vi "PRM - GetParameter.vi"(8 "error in (no error)":errorcluster, 11 "PRM":T1) -> (0 "error out":errorcluster, 3 "PRM OUT":T1, 5 "ParameterString":string)   [LabVIEW 2016]
doc: "Low Level function call. Converts LabVIEW enumeration to xiAPI parameter String."
uses:
  PRM_v2.ctl
  C:/Users/Ries Lab/Documents/Microscope Control from Sheng Account/Microscope-Control/Device Library/Cameras/Ximea/xiLIB_64bit/xiLIB/xiCamLib/API/x64/xiApi.NETX64.dll
  API/x64/xiApi.NETX64.dll
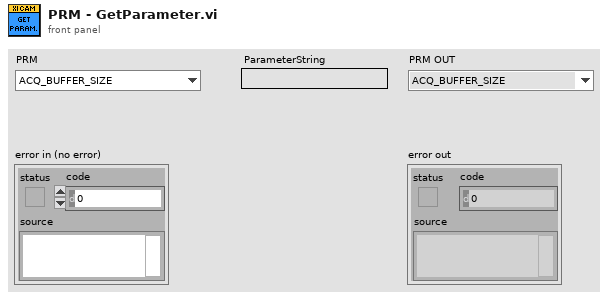
[diagram p1: front panel]
types:
  T1 = typedef "PRM_v2.ctl" = enum16{"ACQ_BUFFER_SIZE", "ACQ_FRAME_BURST_COUNT", "ACQ_TIMING_MODE", "ACQ_TRANSPORT_BUFFER_SIZE", "AE_MAX_LIMIT", "AEAG", "AEAG_LEVEL", "API_VERSION", "AG_MAX_LIMIT", "APPLY_CMS", "AUTO_BANDWIDTH_CALCULATION", "AUTO_WB", "AVAILABLE_BANDWIDTH", "AVAILABLE_BANDWIDTH_MAX", "AVAILABLE_BANDWIDTH_MIN", "BUFFER_POLICY", "BUFFERS_QUEUE_SIZE", "CC_MATRIX_00", "CC_MATRIX_01", "CC_MATRIX_02", "CC_MATRIX_03", "CC_MATRIX_10", "CC_MATRIX_11", "CC_MATRIX_12", "CC_MATRIX_13", "CC_MATRIX_20", "CC_MATRIX_21", "CC_MATRIX_22", "CC_MATRIX_23", "CC_MATRIX_30", "CC_MATRIX_31", "CC_MATRIX_32", "CC_MATRIX_33", "CHIP_TEMP", "CMS", "COLOR_FILTER_ARRAY", "COOLING", "DEBOUNCE_EN", "DEBOUNCE_POL", "DEBOUNCE_T0", "DEBOUNCE_T1", "DEBUG_LEVEL", "DEFAULT_CC_MATRIX", "DEVICE_INSTANCE_PATH", "DEVICE_MODEL_ID", "DEVICE_NAME", "DEVICE_SN", "DEVICE_TYPE", "DEVICE_USER_ID", "DOWNSAMPLING", "DOWNSAMPLING_TYPE", "DRV_VERSION", "EXP_PRIORITY", "EXPOSURE", "EXPOSURE_MAX", "EXPOSURE_MIN", "FFS_FILE_NAME", "FPGA1_VERSION", "FRAMERATE", "FRAMERATE_MAX", "FRAMERATE_MIN", "FREE_FFS_SIZE", "GAIN", "GAIN_MAX", "GAIN_MIN", "GAMMAC", "GAMMAY", "GPI_LEVEL", "GPI_MODE", "GPI_SELECTOR", "GPO_MODE", "GPO_SELECTOR", "HDR", "HDR_T1", "HDR_T2", "HEIGHT", "HEIGHT_MAX", "HEIGHT_MIN", "HOUSE_TEMP", "IMAGE_DATA_FORMAT", "IMAGE_IS_COLOR", "INPUT_CMS_PROFILE", "IS_COOLED", "IS_DEVICE_EXIST", "KNEEPOINT1", "KNEEPOINT2", "LED_MODE", "LED_SELECTOR", "LIMIT_BANDWIDTH", "LIMIT_BANDWIDTH_MAX", "LIMIT_BANDWIDTH_MIN", "LUT_EN", "LUT_INDEX", "LUT_INDEX_MAX", "LUT_INDEX_MIN", "LUT_VALUE", "LUT_VALUE_MAX", "LUT_VALUE_MIN", "MANUAL_WB", "MCU1_VERSION", "MCU2_VERSION", "OFFSET_X", "OFFSET_X_MAX", "OFFSET_X_MIN", "OFFSET_Y", "OFFSET_Y_MAX", "OFFSET_Y_MIN", "OUTPUT_CMS_PROFILE", "OUTPUT_DATA_BIT_DEPTH", "OUTPUT_DATA_PACKING", "READ_FILE_FFS", "RECENT_FRAME", "SENSOR_DATA_BIT_DEPTH", "SENSOR_MODE", "SENSOR_TAPS", "SHARPNESS", "SHUTTER_TYPE", "TARGET_TEMP", "TRG_DELAY", "TRG_SELECTOR", "TRG_SOFTWARE", "TRG_SOURCE", "USED_FFS_SIZE", "WB_KB", "WB_KG", "WB_KR", "WIDTH", "WIDTH_MAX", "WIDTH_MIN", "WRITE_FILE_FFS", "ACQ_BUFFER_SIZE_UNIT", "ACQ_TRANSPORT_BUFFER_COMMIT", "AEAG_ROI_HEIGHT", "AEAG_ROI_OFFSET_X", "AEAG_ROU_OFFSET_Y", "AEAG_ROI_WIDTH", "API_CONTEXT_LIST", "BINNING_HORIZONTAL", "BINNING_SELECTOR", "BINNING_VERTICAL", "COLUMN_FPN_CORRECTION", "COUNTER_SELECTOR", "COUNTER_VALUE", "DECIMATION_HORIZONTAL", "DECIMATION_SELECTOR", "DECIMATION_VERTICAL", "DEVICE_ID", "DEVICE_LOCATION_PATH", "DEVICE_MANIFEST", "DEVICE_RESET", "DEVICE_SENS_SN", "EXPOSURE_BURST_COUNT", "FFS_ACCESS_KEY", "GAIN_SELECTOR", "HW_REVISION", "IMAGE_BLACK_LEVEL", "IMAGE_DATA_BIT_DEPTH", "IMAGE_DATA_FORMAT_RGB32_ALPHA", "IMAGE_PAYLOAD_SIZE", "LENS_APERTURE_VALUE", "LENS_FEATURE", "LENS_FEATURE_SELECTOR", "LENS_FOCAL_LENGTH", "LENS_FOCUS_DISTANCE", "LENS_FOCUS_MOVE", "LENS_FOCUS_MOVEMENT_VALUE", "LENS_MODE", "OUTPUT_DATA_PACKING_TYPE", "SENSOR_CLOCK_FREQ_HZ", "SENSOR_CLOCK_FREQ_INDEX", "SENSOR_FEATURE_SELECTOR", "SENSOR_FEATURE_VALUE", "SENSOR_OUTPUT_CHANNEL_COUNT", "TRANSPORT_PIXEL_FORMAT", "TS_RST_MODE", "TS_RST_SOURCE", "SENS_DEFECTS_CORR_LIST_SELECTOR", "SENS_DEFECTS_CORR", "SENS_DEFECTS_CORR_LIST_CONTENT", "DEVICE_UNIT_SELECTOR", "DEVICE_UNIT_REGISTER_SELECTOR", "DEVICE_UNIT_REGISTER_VALUE"}
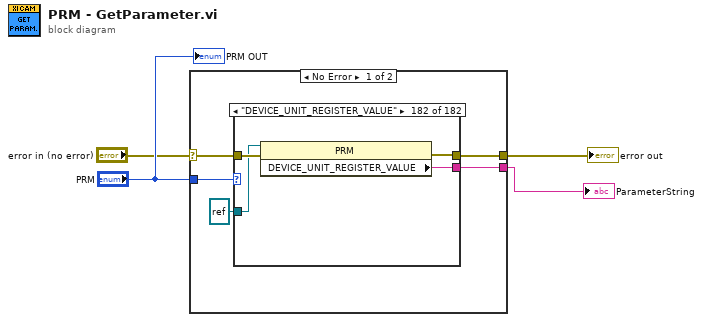
[diagram p0: block diagram]
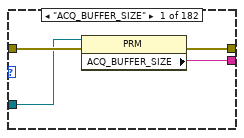
[diagram p2: hidden frame]
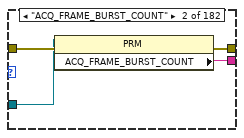
[diagram p3: hidden frame]
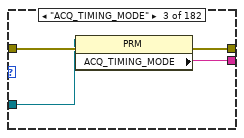
[diagram p4: hidden frame]
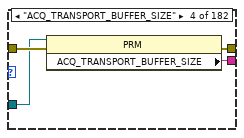
[diagram p5: hidden frame]
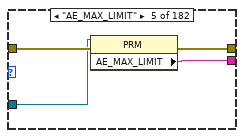
[diagram p6: hidden frame]
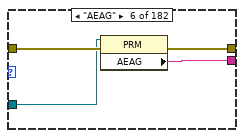
[diagram p7: hidden frame]
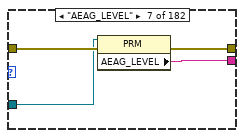
[diagram p8: hidden frame]
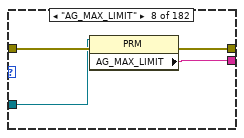
[diagram p9: hidden frame]
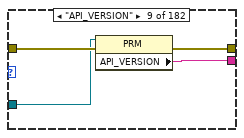
[diagram p10: hidden frame]
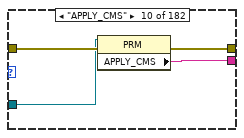
[diagram p11: hidden frame]
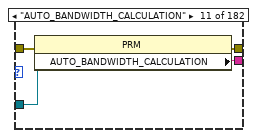
[diagram p12: hidden frame]
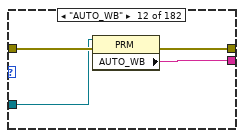
[diagram p13: hidden frame]
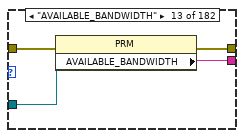
[diagram p14: hidden frame]
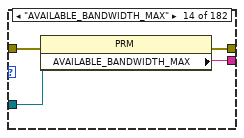
[diagram p15: hidden frame]
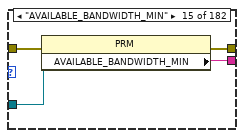
[diagram p16: hidden frame]
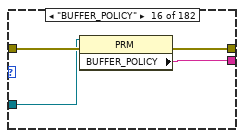
[diagram p17: hidden frame]
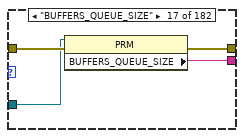
[diagram p18: hidden frame]
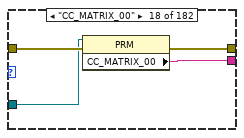
[diagram p19: hidden frame]
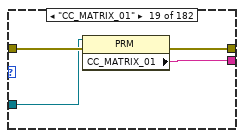
[diagram p20: hidden frame]
diagram:
  n1 = case shown="No Error" "error in (no error)" {
    selector: "error in (no error)" -> [w8 w738]
    tunnel: "PRM" -> [w9 _]
    tunnel: [w7 _] -> w1
    tunnel: [w6 w738] -> w2
    frame No Error {
      n2 = case shown="\"DEVICE_UNIT_REGISTER_VALUE\"" w9 {
        tunnel: w8 -> [w13 w17 w21 w25 w29 w33 w37 w41 w45 w49 w53 w57 w61 w65 w69 w73 w77 w81 w85 w89 w93 w97 w101 w105 w109 w113 w117 w121 w125 w129 w133 w137 w141 w145 w149 w153 w157 w161 w165 w169 w173 w177 w181 w185 w189 w193 w197 w201 w205 w209 w213 w217 w221 w225 w229 w233 w237 w241 w245 w249 w253 w257 w261 w265 w269 w273 w277 w281 w285 w289 w293 w297 w301 w305 w309 w313 w317 w321 w325 w329 w333 w337 w341 w345 w349 w353 w357 w361 w365 w369 w373 w377 w381 w385 w389 w393 w397 w401 w405 w409 w413 w417 w421 w425 w429 w433 w437 w441 w445 w449 w453 w457 w461 w465 w469 w473 w477 w481 w485 w489 w493 w497 w501 w505 w509 w513 w517 w521 w525 w529 w532 w536 w540 w544 w548 w552 w556 w560 w564 w568 w572 w576 w580 w584 w588 w592 w596 w600 w604 w608 w612 w616 w620 w624 w628 w632 w636 w640 w644 w648 w652 w656 w660 w664 w668 w672 w676 w680 w684 w688 w692 w696 w700 w704 w708 w712 w715 w721 w725 w729 w733 w737]
        tunnel: [w12 w16 w20 w24 w28 w32 w36 w40 w44 w48 w52 w56 w60 w64 w68 w72 w76 w80 w84 w88 w92 w96 w100 w104 w108 w112 w116 w120 w124 w128 w132 w136 w140 w144 w148 w152 w156 w160 w164 w168 w172 w176 w180 w184 w188 w192 w196 w200 w204 w208 w212 w216 w220 w224 w228 w232 w236 w240 w244 w248 w252 w256 w260 w264 w268 w272 w276 w280 w284 w288 w292 w296 w300 w304 w308 w312 w316 w320 w324 w328 w332 w336 w340 w344 w348 w352 w356 w360 w364 w368 w372 w376 w380 w384 w388 w392 w396 w400 w404 w408 w412 w416 w420 w424 w428 w432 w436 w440 w444 w448 w452 w456 w460 w464 w468 w472 w476 w480 w484 w488 w492 w496 w500 w504 w508 w512 w516 w520 w524 w528 w530 w534 w538 w542 w546 w550 w554 w558 w562 w566 w570 w574 w578 w582 w586 w590 w594 w598 w602 w606 w610 w614 w618 w622 w626 w630 w634 w638 w642 w646 w650 w654 w658 w662 w666 w670 w674 w678 w682 w686 w690 w694 w698 w702 w706 w710 w717 w719 w723 w726 w730 w734] -> w7
        tunnel: [w11 w15 w19 w23 w27 w31 w35 w39 w43 w47 w51 w55 w59 w63 w67 w71 w75 w79 w83 w87 w91 w95 w99 w103 w107 w111 w115 w119 w123 w127 w131 w135 w139 w143 w147 w151 w155 w159 w163 w167 w171 w175 w179 w183 w187 w191 w195 w199 w203 w207 w211 w215 w219 w223 w227 w231 w235 w239 w243 w247 w251 w255 w259 w263 w267 w271 w275 w279 w283 w287 w291 w295 w299 w303 w307 w311 w315 w319 w323 w327 w331 w335 w339 w343 w347 w351 w355 w359 w363 w367 w371 w375 w379 w383 w387 w391 w395 w399 w403 w407 w411 w415 w419 w423 w427 w431 w435 w439 w443 w447 w451 w455 w459 w463 w467 w471 w475 w479 w483 w487 w491 w495 w499 w503 w507 w511 w515 w519 w523 w527 w531 w535 w539 w543 w547 w551 w555 w559 w563 w567 w571 w575 w579 w583 w587 w591 w595 w599 w603 w607 w611 w615 w619 w623 w627 w631 w635 w639 w643 w647 w651 w655 w659 w663 w667 w671 w675 w679 w683 w687 w691 w695 w699 w703 w707 w711 w716 w720 w724 w727 w731 w735] -> w6
        tunnel: refnum<k24> refnum ("reference") -> [w10 w14 w18 w22 w26 w30 w34 w38 w42 w46 w50 w54 w58 w62 w66 w70 w74 w78 w82 w86 w90 w94 w98 w102 w106 w110 w114 w118 w122 w126 w130 w134 w138 w142 w146 w150 w154 w158 w162 w166 w170 w174 w178 w182 w186 w190 w194 w198 w202 w206 w210 w214 w218 w222 w226 w230 w234 w238 w242 w246 w250 w254 w258 w262 w266 w270 w274 w278 w282 w286 w290 w294 w298 w302 w306 w310 w314 w318 w322 w326 w330 w334 w338 w342 w346 w350 w354 w358 w362 w366 w370 w374 w378 w382 w386 w390 w394 w398 w402 w406 w410 w414 w418 w422 w426 w430 w434 w438 w442 w446 w450 w454 w458 w462 w466 w470 w474 w478 w482 w486 w490 w494 w498 w502 w506 w510 w514 w518 w522 w526 w533 w537 w541 w545 w549 w553 w557 w561 w565 w569 w573 w577 w581 w585 w589 w593 w597 w601 w605 w609 w613 w617 w621 w625 w629 w633 w637 w641 w645 w649 w653 w657 w661 w665 w669 w673 w677 w681 w685 w689 w693 w697 w701 w705 w709 w713 w714 w718 w722 w728 w732 w736]
        frame "ACQ_BUFFER_SIZE" {
          n3 = property class="PRM"(reference=w10, error in=w13) -> (error out=w11:errorcluster, "ACQ_BUFFER_SIZE"=w12:string)  [unwired: 1 out]
        }
        frame "ACQ_FRAME_BURST_COUNT" {
          n4 = property class="PRM"(reference=w14, error in=w17) -> (error out=w15:errorcluster, "ACQ_FRAME_BURST_COUNT"=w16:string)  [unwired: 1 out]
        }
        frame "ACQ_TIMING_MODE" {
          n5 = property class="PRM"(reference=w18, error in=w21) -> (error out=w19:errorcluster, "ACQ_TIMING_MODE"=w20:string)  [unwired: 1 out]
        }
        frame "ACQ_TRANSPORT_BUFFER_SIZE" {
          n6 = property class="PRM"(reference=w22, error in=w25) -> (error out=w23:errorcluster, "ACQ_TRANSPORT_BUFFER_SIZE"=w24:string)  [unwired: 1 out]
        }
        frame "AE_MAX_LIMIT" {
          n7 = property class="PRM"(reference=w26, error in=w29) -> (error out=w27:errorcluster, "AE_MAX_LIMIT"=w28:string)  [unwired: 1 out]
        }
        frame "AEAG" {
          n8 = property class="PRM"(reference=w30, error in=w33) -> (error out=w31:errorcluster, "AEAG"=w32:string)  [unwired: 1 out]
        }
        frame "AEAG_LEVEL" {
          n9 = property class="PRM"(reference=w34, error in=w37) -> (error out=w35:errorcluster, "AEAG_LEVEL"=w36:string)  [unwired: 1 out]
        }
        frame "AG_MAX_LIMIT" {
          n10 = property class="PRM"(reference=w38, error in=w41) -> (error out=w39:errorcluster, "AG_MAX_LIMIT"=w40:string)  [unwired: 1 out]
        }
        frame "API_VERSION" {
          n11 = property class="PRM"(reference=w42, error in=w45) -> (error out=w43:errorcluster, "API_VERSION"=w44:string)  [unwired: 1 out]
        }
        frame "APPLY_CMS" {
          n12 = property class="PRM"(reference=w46, error in=w49) -> (error out=w47:errorcluster, "APPLY_CMS"=w48:string)  [unwired: 1 out]
        }
        frame "AUTO_BANDWIDTH_CALCULATION" {
          n13 = property class="PRM"(reference=w50, error in=w53) -> (error out=w51:errorcluster, "AUTO_BANDWIDTH_CALCULATION"=w52:string)  [unwired: 1 out]
        }
        frame "AUTO_WB" {
          n14 = property class="PRM"(reference=w54, error in=w57) -> (error out=w55:errorcluster, "AUTO_WB"=w56:string)  [unwired: 1 out]
        }
        frame "AVAILABLE_BANDWIDTH" {
          n15 = property class="PRM"(reference=w58, error in=w61) -> (error out=w59:errorcluster, "AVAILABLE_BANDWIDTH"=w60:string)  [unwired: 1 out]
        }
        frame "AVAILABLE_BANDWIDTH_MAX" {
          n16 = property class="PRM"(reference=w62, error in=w65) -> (error out=w63:errorcluster, "AVAILABLE_BANDWIDTH_MAX"=w64:string)  [unwired: 1 out]
        }
        frame "AVAILABLE_BANDWIDTH_MIN" {
          n17 = property class="PRM"(reference=w66, error in=w69) -> (error out=w67:errorcluster, "AVAILABLE_BANDWIDTH_MIN"=w68:string)  [unwired: 1 out]
        }
        frame "BUFFER_POLICY" {
          n18 = property class="PRM"(reference=w70, error in=w73) -> (error out=w71:errorcluster, "BUFFER_POLICY"=w72:string)  [unwired: 1 out]
        }
        frame "BUFFERS_QUEUE_SIZE" {
          n19 = property class="PRM"(reference=w74, error in=w77) -> (error out=w75:errorcluster, "BUFFERS_QUEUE_SIZE"=w76:string)  [unwired: 1 out]
        }
        frame "CC_MATRIX_00" {
          n20 = property class="PRM"(reference=w78, error in=w81) -> (error out=w79:errorcluster, "CC_MATRIX_00"=w80:string)  [unwired: 1 out]
        }
        frame "CC_MATRIX_01" {
          n21 = property class="PRM"(reference=w82, error in=w85) -> (error out=w83:errorcluster, "CC_MATRIX_01"=w84:string)  [unwired: 1 out]
        }
        frame "CC_MATRIX_02" {
          n22 = property class="PRM"(reference=w86, error in=w89) -> (error out=w87:errorcluster, "CC_MATRIX_02"=w88:string)  [unwired: 1 out]
        }
        frame "CC_MATRIX_03" {
          n23 = property class="PRM"(reference=w90, error in=w93) -> (error out=w91:errorcluster, "CC_MATRIX_03"=w92:string)  [unwired: 1 out]
        }
        frame "CC_MATRIX_10" {
          n24 = property class="PRM"(reference=w94, error in=w97) -> (error out=w95:errorcluster, "CC_MATRIX_10"=w96:string)  [unwired: 1 out]
        }
        frame "CC_MATRIX_11" {
          n25 = property class="PRM"(reference=w98, error in=w101) -> (error out=w99:errorcluster, "CC_MATRIX_11"=w100:string)  [unwired: 1 out]
        }
        frame "CC_MATRIX_12" {
          n26 = property class="PRM"(reference=w102, error in=w105) -> (error out=w103:errorcluster, "CC_MATRIX_12"=w104:string)  [unwired: 1 out]
        }
        frame "CC_MATRIX_13" {
          n27 = property class="PRM"(reference=w106, error in=w109) -> (error out=w107:errorcluster, "CC_MATRIX_13"=w108:string)  [unwired: 1 out]
        }
        frame "CC_MATRIX_20" {
          n28 = property class="PRM"(reference=w110, error in=w113) -> (error out=w111:errorcluster, "CC_MATRIX_20"=w112:string)  [unwired: 1 out]
        }
        frame "CC_MATRIX_21" {
          n29 = property class="PRM"(reference=w114, error in=w117) -> (error out=w115:errorcluster, "CC_MATRIX_21"=w116:string)  [unwired: 1 out]
        }
        frame "CC_MATRIX_22" {
          n30 = property class="PRM"(reference=w118, error in=w121) -> (error out=w119:errorcluster, "CC_MATRIX_22"=w120:string)  [unwired: 1 out]
        }
        frame "CC_MATRIX_23" {
          n31 = property class="PRM"(reference=w122, error in=w125) -> (error out=w123:errorcluster, "CC_MATRIX_23"=w124:string)  [unwired: 1 out]
        }
        frame "CC_MATRIX_30" {
          n32 = property class="PRM"(reference=w126, error in=w129) -> (error out=w127:errorcluster, "CC_MATRIX_30"=w128:string)  [unwired: 1 out]
        }
        frame "CC_MATRIX_31" {
          n33 = property class="PRM"(reference=w130, error in=w133) -> (error out=w131:errorcluster, "CC_MATRIX_31"=w132:string)  [unwired: 1 out]
        }
        frame "CC_MATRIX_32" {
          n34 = property class="PRM"(reference=w134, error in=w137) -> (error out=w135:errorcluster, "CC_MATRIX_32"=w136:string)  [unwired: 1 out]
        }
        frame "CC_MATRIX_33" {
          n35 = property class="PRM"(reference=w138, error in=w141) -> (error out=w139:errorcluster, "CC_MATRIX_33"=w140:string)  [unwired: 1 out]
        }
        frame "CHIP_TEMP" {
          n36 = property class="PRM"(reference=w142, error in=w145) -> (error out=w143:errorcluster, "CHIP_TEMP"=w144:string)  [unwired: 1 out]
        }
        frame "CMS" {
          n37 = property class="PRM"(reference=w146, error in=w149) -> (error out=w147:errorcluster, "CMS"=w148:string)  [unwired: 1 out]
        }
        frame "COLOR_FILTER_ARRAY" {
          n38 = property class="PRM"(reference=w150, error in=w153) -> (error out=w151:errorcluster, "COLOR_FILTER_ARRAY"=w152:string)  [unwired: 1 out]
        }
        frame "COOLING" {
          n39 = property class="PRM"(reference=w154, error in=w157) -> (error out=w155:errorcluster, "COOLING"=w156:string)  [unwired: 1 out]
        }
        frame "DEBOUNCE_EN" {
          n40 = property class="PRM"(reference=w158, error in=w161) -> (error out=w159:errorcluster, "DEBOUNCE_EN"=w160:string)  [unwired: 1 out]
        }
        frame "DEBOUNCE_POL" {
          n41 = property class="PRM"(reference=w162, error in=w165) -> (error out=w163:errorcluster, "DEBOUNCE_POL"=w164:string)  [unwired: 1 out]
        }
        frame "DEBOUNCE_T0" {
          n42 = property class="PRM"(reference=w166, error in=w169) -> (error out=w167:errorcluster, "DEBOUNCE_T0"=w168:string)  [unwired: 1 out]
        }
        frame "DEBOUNCE_T1" {
          n43 = property class="PRM"(reference=w170, error in=w173) -> (error out=w171:errorcluster, "DEBOUNCE_T1"=w172:string)  [unwired: 1 out]
        }
        frame "DEBUG_LEVEL" {
          n44 = property class="PRM"(reference=w174, error in=w177) -> (error out=w175:errorcluster, "DEBUG_LEVEL"=w176:string)  [unwired: 1 out]
        }
        frame "DEFAULT_CC_MATRIX" {
          n45 = property class="PRM"(reference=w178, error in=w181) -> (error out=w179:errorcluster, "DEFAULT_CC_MATRIX"=w180:string)  [unwired: 1 out]
        }
        frame "DEVICE_INSTANCE_PATH" {
          n46 = property class="PRM"(reference=w182, error in=w185) -> (error out=w183:errorcluster, "DEVICE_INSTANCE_PATH"=w184:string)  [unwired: 1 out]
        }
        frame "DEVICE_MODEL_ID" {
          n47 = property class="PRM"(reference=w186, error in=w189) -> (error out=w187:errorcluster, "DEVICE_MODEL_ID"=w188:string)  [unwired: 1 out]
        }
        frame "DEVICE_NAME" {
          n48 = property class="PRM"(reference=w190, error in=w193) -> (error out=w191:errorcluster, "DEVICE_NAME"=w192:string)  [unwired: 1 out]
        }
        frame "DEVICE_SN" {
          n49 = property class="PRM"(reference=w194, error in=w197) -> (error out=w195:errorcluster, "DEVICE_SN"=w196:string)  [unwired: 1 out]
        }
        frame "DEVICE_TYPE" {
          n50 = property class="PRM"(reference=w198, error in=w201) -> (error out=w199:errorcluster, "DEVICE_TYPE"=w200:string)  [unwired: 1 out]
        }
        frame "DEVICE_USER_ID" {
          n51 = property class="PRM"(reference=w202, error in=w205) -> (error out=w203:errorcluster, "DEVICE_USER_ID"=w204:string)  [unwired: 1 out]
        }
        frame "DOWNSAMPLING" {
          n52 = property class="PRM"(reference=w206, error in=w209) -> (error out=w207:errorcluster, "DOWNSAMPLING"=w208:string)  [unwired: 1 out]
        }
        frame "DOWNSAMPLING_TYPE" {
          n53 = property class="PRM"(reference=w210, error in=w213) -> (error out=w211:errorcluster, "DOWNSAMPLING_TYPE"=w212:string)  [unwired: 1 out]
        }
        frame "DRV_VERSION" {
          n54 = property class="PRM"(reference=w214, error in=w217) -> (error out=w215:errorcluster, "DRV_VERSION"=w216:string)  [unwired: 1 out]
        }
        frame "EXP_PRIORITY" {
          n55 = property class="PRM"(reference=w218, error in=w221) -> (error out=w219:errorcluster, "EXP_PRIORITY"=w220:string)  [unwired: 1 out]
        }
        frame "EXPOSURE" {
          n56 = property class="PRM"(reference=w222, error in=w225) -> (error out=w223:errorcluster, "EXPOSURE"=w224:string)  [unwired: 1 out]
        }
        frame "EXPOSURE_MAX" {
          n57 = property class="PRM"(reference=w226, error in=w229) -> (error out=w227:errorcluster, "EXPOSURE_MAX"=w228:string)  [unwired: 1 out]
        }
        frame "EXPOSURE_MIN" {
          n58 = property class="PRM"(reference=w230, error in=w233) -> (error out=w231:errorcluster, "EXPOSURE_MIN"=w232:string)  [unwired: 1 out]
        }
        frame "FFS_FILE_NAME" {
          n59 = property class="PRM"(reference=w234, error in=w237) -> (error out=w235:errorcluster, "FFS_FILE_NAME"=w236:string)  [unwired: 1 out]
        }
        frame "FPGA1_VERSION" {
          n60 = property class="PRM"(reference=w238, error in=w241) -> (error out=w239:errorcluster, "FPGA1_VERSION"=w240:string)  [unwired: 1 out]
        }
        frame "FRAMERATE" {
          n61 = property class="PRM"(reference=w242, error in=w245) -> (error out=w243:errorcluster, "FRAMERATE"=w244:string)  [unwired: 1 out]
        }
        frame "FRAMERATE_MAX" {
          n62 = property class="PRM"(reference=w246, error in=w249) -> (error out=w247:errorcluster, "FRAMERATE_MAX"=w248:string)  [unwired: 1 out]
        }
        frame "FRAMERATE_MIN" {
          n63 = property class="PRM"(reference=w250, error in=w253) -> (error out=w251:errorcluster, "FRAMERATE_MIN"=w252:string)  [unwired: 1 out]
        }
        frame "FREE_FFS_SIZE" {
          n64 = property class="PRM"(reference=w254, error in=w257) -> (error out=w255:errorcluster, "FREE_FFS_SIZE"=w256:string)  [unwired: 1 out]
        }
        frame "GAIN" {
          n65 = property class="PRM"(reference=w258, error in=w261) -> (error out=w259:errorcluster, "GAIN"=w260:string)  [unwired: 1 out]
        }
        frame "GAIN_MAX" {
          n66 = property class="PRM"(reference=w262, error in=w265) -> (error out=w263:errorcluster, "GAIN_MAX"=w264:string)  [unwired: 1 out]
        }
        frame "GAIN_MIN" {
          n67 = property class="PRM"(reference=w266, error in=w269) -> (error out=w267:errorcluster, "GAIN_MIN"=w268:string)  [unwired: 1 out]
        }
        frame "GAMMAC" {
          n68 = property class="PRM"(reference=w270, error in=w273) -> (error out=w271:errorcluster, "GAMMAC"=w272:string)  [unwired: 1 out]
        }
        frame "GAMMAY" {
          n69 = property class="PRM"(reference=w274, error in=w277) -> (error out=w275:errorcluster, "GAMMAY"=w276:string)  [unwired: 1 out]
        }
        frame "GPI_LEVEL" {
          n70 = property class="PRM"(reference=w278, error in=w281) -> (error out=w279:errorcluster, "GPI_LEVEL"=w280:string)  [unwired: 1 out]
        }
        frame "GPI_MODE" {
          n71 = property class="PRM"(reference=w282, error in=w285) -> (error out=w283:errorcluster, "GPI_MODE"=w284:string)  [unwired: 1 out]
        }
        frame "GPI_SELECTOR" {
          n72 = property class="PRM"(reference=w286, error in=w289) -> (error out=w287:errorcluster, "GPI_SELECTOR"=w288:string)  [unwired: 1 out]
        }
        frame "GPO_MODE" {
          n73 = property class="PRM"(reference=w290, error in=w293) -> (error out=w291:errorcluster, "GPO_MODE"=w292:string)  [unwired: 1 out]
        }
        frame "GPO_SELECTOR" {
          n74 = property class="PRM"(reference=w294, error in=w297) -> (error out=w295:errorcluster, "GPO_SELECTOR"=w296:string)  [unwired: 1 out]
        }
        frame "HDR" {
          n75 = property class="PRM"(reference=w298, error in=w301) -> (error out=w299:errorcluster, "HDR"=w300:string)  [unwired: 1 out]
        }
        frame "HDR_T1" {
          n76 = property class="PRM"(reference=w302, error in=w305) -> (error out=w303:errorcluster, "HDR_T1"=w304:string)  [unwired: 1 out]
        }
        frame "HDR_T2" {
          n77 = property class="PRM"(reference=w306, error in=w309) -> (error out=w307:errorcluster, "HDR_T2"=w308:string)  [unwired: 1 out]
        }
        frame "HEIGHT" {
          n78 = property class="PRM"(reference=w310, error in=w313) -> (error out=w311:errorcluster, "HEIGHT"=w312:string)  [unwired: 1 out]
        }
        frame "HEIGHT_MAX" {
          n79 = property class="PRM"(reference=w314, error in=w317) -> (error out=w315:errorcluster, "HEIGHT_MAX"=w316:string)  [unwired: 1 out]
        }
        frame "HEIGHT_MIN" {
          n80 = property class="PRM"(reference=w318, error in=w321) -> (error out=w319:errorcluster, "HEIGHT_MIN"=w320:string)  [unwired: 1 out]
        }
        frame "HOUSE_TEMP" {
          n81 = property class="PRM"(reference=w322, error in=w325) -> (error out=w323:errorcluster, "HOUS_TEMP"=w324:string)  [unwired: 1 out]
        }
        frame "IMAGE_DATA_FORMAT" {
          n82 = property class="PRM"(reference=w326, error in=w329) -> (error out=w327:errorcluster, "IMAGE_DATA_FORMAT"=w328:string)  [unwired: 1 out]
        }
        frame "IMAGE_IS_COLOR" {
          n83 = property class="PRM"(reference=w330, error in=w333) -> (error out=w331:errorcluster, "IMAGE_IS_COLOR"=w332:string)  [unwired: 1 out]
        }
        frame "INPUT_CMS_PROFILE" {
          n84 = property class="PRM"(reference=w334, error in=w337) -> (error out=w335:errorcluster, "INPUT_CMS_PROFILE"=w336:string)  [unwired: 1 out]
        }
        frame "IS_COOLED" {
          n85 = property class="PRM"(reference=w338, error in=w341) -> (error out=w339:errorcluster, "IS_COOLED"=w340:string)  [unwired: 1 out]
        }
        frame "IS_DEVICE_EXIST" {
          n86 = property class="PRM"(reference=w342, error in=w345) -> (error out=w343:errorcluster, "IS_DEVICE_EXIST"=w344:string)  [unwired: 1 out]
        }
        frame "KNEEPOINT1" {
          n87 = property class="PRM"(reference=w346, error in=w349) -> (error out=w347:errorcluster, "KNEEPOINT1"=w348:string)  [unwired: 1 out]
        }
        frame "KNEEPOINT2" {
          n88 = property class="PRM"(reference=w350, error in=w353) -> (error out=w351:errorcluster, "KNEEPOINT2"=w352:string)  [unwired: 1 out]
        }
        frame "LED_MODE" {
          n89 = property class="PRM"(reference=w354, error in=w357) -> (error out=w355:errorcluster, "LED_MODE"=w356:string)  [unwired: 1 out]
        }
        frame "LED_SELECTOR" {
          n90 = property class="PRM"(reference=w358, error in=w361) -> (error out=w359:errorcluster, "LED_SELECTOR"=w360:string)  [unwired: 1 out]
        }
        frame "LIMIT_BANDWIDTH" {
          n91 = property class="PRM"(reference=w362, error in=w365) -> (error out=w363:errorcluster, "LIMIT_BANDWIDTH"=w364:string)  [unwired: 1 out]
        }
        frame "LIMIT_BANDWIDTH_MAX" {
          n92 = property class="PRM"(reference=w366, error in=w369) -> (error out=w367:errorcluster, "LIMIT_BANDWIDTH_MAX"=w368:string)  [unwired: 1 out]
        }
        frame "LIMIT_BANDWIDTH_MIN" {
          n93 = property class="PRM"(reference=w370, error in=w373) -> (error out=w371:errorcluster, "LIMIT_BANDWIDTH_MIN"=w372:string)  [unwired: 1 out]
        }
        frame "LUT_EN" {
          n94 = property class="PRM"(reference=w374, error in=w377) -> (error out=w375:errorcluster, "LUT_EN"=w376:string)  [unwired: 1 out]
        }
        frame "LUT_INDEX" {
          n95 = property class="PRM"(reference=w378, error in=w381) -> (error out=w379:errorcluster, "LUT_INDEX"=w380:string)  [unwired: 1 out]
        }
        frame "LUT_INDEX_MAX" {
          n96 = property class="PRM"(reference=w382, error in=w385) -> (error out=w383:errorcluster, "LUT_INDEX_MAX"=w384:string)  [unwired: 1 out]
        }
        frame "LUT_INDEX_MIN" {
          n97 = property class="PRM"(reference=w386, error in=w389) -> (error out=w387:errorcluster, "LUT_INDEX_MIN"=w388:string)  [unwired: 1 out]
        }
        frame "LUT_VALUE" {
          n98 = property class="PRM"(reference=w390, error in=w393) -> (error out=w391:errorcluster, "LUT_VALUE"=w392:string)  [unwired: 1 out]
        }
        frame "LUT_VALUE_MAX" {
          n99 = property class="PRM"(reference=w394, error in=w397) -> (error out=w395:errorcluster, "LUT_VALUE_MAX"=w396:string)  [unwired: 1 out]
        }
        frame "LUT_VALUE_MIN" {
          n100 = property class="PRM"(reference=w398, error in=w401) -> (error out=w399:errorcluster, "LUT_VALUE_MIN"=w400:string)  [unwired: 1 out]
        }
        frame "MANUAL_WB" {
          n101 = property class="PRM"(reference=w402, error in=w405) -> (error out=w403:errorcluster, "MANUAL_WB"=w404:string)  [unwired: 1 out]
        }
        frame "MCU1_VERSION" {
          n102 = property class="PRM"(reference=w406, error in=w409) -> (error out=w407:errorcluster, "MCU1_VERSION"=w408:string)  [unwired: 1 out]
        }
        frame "MCU2_VERSION" {
          n103 = property class="PRM"(reference=w410, error in=w413) -> (error out=w411:errorcluster, "MCU2_VERSION"=w412:string)  [unwired: 1 out]
        }
        frame "OFFSET_X" {
          n104 = property class="PRM"(reference=w414, error in=w417) -> (error out=w415:errorcluster, "OFFSET_X"=w416:string)  [unwired: 1 out]
        }
        frame "OFFSET_X_MAX" {
          n105 = property class="PRM"(reference=w418, error in=w421) -> (error out=w419:errorcluster, "OFFSET_X_MAX"=w420:string)  [unwired: 1 out]
        }
        frame "OFFSET_X_MIN" {
          n106 = property class="PRM"(reference=w422, error in=w425) -> (error out=w423:errorcluster, "OFFSET_X_MIN"=w424:string)  [unwired: 1 out]
        }
        frame "OFFSET_Y" {
          n107 = property class="PRM"(reference=w426, error in=w429) -> (error out=w427:errorcluster, "OFFSET_Y"=w428:string)  [unwired: 1 out]
        }
        frame "OFFSET_Y_MAX" {
          n108 = property class="PRM"(reference=w430, error in=w433) -> (error out=w431:errorcluster, "OFFSET_Y_MAX"=w432:string)  [unwired: 1 out]
        }
        frame "OFFSET_Y_MIN" {
          n109 = property class="PRM"(reference=w434, error in=w437) -> (error out=w435:errorcluster, "OFFSET_Y_MIN"=w436:string)  [unwired: 1 out]
        }
        frame "OUTPUT_CMS_PROFILE" {
          n110 = property class="PRM"(reference=w438, error in=w441) -> (error out=w439:errorcluster, "OUTPUT_CMS_PROFILE"=w440:string)  [unwired: 1 out]
        }
        frame "OUTPUT_DATA_BIT_DEPTH" {
          n111 = property class="PRM"(reference=w442, error in=w445) -> (error out=w443:errorcluster, "OUTPUT_DATA_BIT_DEPTH"=w444:string)  [unwired: 1 out]
        }
        frame "OUTPUT_DATA_PACKING" {
          n112 = property class="PRM"(reference=w446, error in=w449) -> (error out=w447:errorcluster, "OUTPUT_DATA_PACKING"=w448:string)  [unwired: 1 out]
        }
        frame "READ_FILE_FFS" {
          n113 = property class="PRM"(reference=w450, error in=w453) -> (error out=w451:errorcluster, "READ_FILE_FFS"=w452:string)  [unwired: 1 out]
        }
        frame "RECENT_FRAME" {
          n114 = property class="PRM"(reference=w454, error in=w457) -> (error out=w455:errorcluster, "RECENT_FRAME"=w456:string)  [unwired: 1 out]
        }
        frame "SENSOR_DATA_BIT_DEPTH" {
          n115 = property class="PRM"(reference=w458, error in=w461) -> (error out=w459:errorcluster, "SENSOR_DATA_BIT_DEPTH"=w460:string)  [unwired: 1 out]
        }
        frame "SENSOR_MODE" {
          n116 = property class="PRM"(reference=w462, error in=w465) -> (error out=w463:errorcluster, "SENSOR_MODE"=w464:string)  [unwired: 1 out]
        }
        frame "SENSOR_TAPS" {
          n117 = property class="PRM"(reference=w466, error in=w469) -> (error out=w467:errorcluster, "SENSOR_TAPS"=w468:string)  [unwired: 1 out]
        }
        frame "SHARPNESS" {
          n118 = property class="PRM"(reference=w470, error in=w473) -> (error out=w471:errorcluster, "SHARPNESS"=w472:string)  [unwired: 1 out]
        }
        frame "SHUTTER_TYPE" {
          n119 = property class="PRM"(reference=w474, error in=w477) -> (error out=w475:errorcluster, "SHUTTER_TYPE"=w476:string)  [unwired: 1 out]
        }
        frame "TARGET_TEMP" {
          n120 = property class="PRM"(reference=w478, error in=w481) -> (error out=w479:errorcluster, "TARGET_TEMP"=w480:string)  [unwired: 1 out]
        }
        frame "TRG_DELAY" {
          n121 = property class="PRM"(reference=w482, error in=w485) -> (error out=w483:errorcluster, "TRG_DELAY"=w484:string)  [unwired: 1 out]
        }
        frame "TRG_SELECTOR" {
          n122 = property class="PRM"(reference=w486, error in=w489) -> (error out=w487:errorcluster, "TRG_SELECTOR"=w488:string)  [unwired: 1 out]
        }
        frame "TRG_SOFTWARE" {
          n123 = property class="PRM"(reference=w490, error in=w493) -> (error out=w491:errorcluster, "TRG_SOFTWARE"=w492:string)  [unwired: 1 out]
        }
        frame "TRG_SOURCE" {
          n124 = property class="PRM"(reference=w494, error in=w497) -> (error out=w495:errorcluster, "TRG_SOURCE"=w496:string)  [unwired: 1 out]
        }
        frame "USED_FFS_SIZE" {
          n125 = property class="PRM"(reference=w498, error in=w501) -> (error out=w499:errorcluster, "USED_FFS_SIZE"=w500:string)  [unwired: 1 out]
        }
        frame "WB_KB" {
          n126 = property class="PRM"(reference=w502, error in=w505) -> (error out=w503:errorcluster, "WB_KB"=w504:string)  [unwired: 1 out]
        }
        frame "WB_KG" {
          n127 = property class="PRM"(reference=w506, error in=w509) -> (error out=w507:errorcluster, "WB_KG"=w508:string)  [unwired: 1 out]
        }
        frame "WB_KR" {
          n128 = property class="PRM"(reference=w510, error in=w513) -> (error out=w511:errorcluster, "WB_KR"=w512:string)  [unwired: 1 out]
        }
        frame "WIDTH" {
          n129 = property class="PRM"(reference=w514, error in=w517) -> (error out=w515:errorcluster, "WIDTH"=w516:string)  [unwired: 1 out]
        }
        frame "WIDTH_MAX" {
          n130 = property class="PRM"(reference=w518, error in=w521) -> (error out=w519:errorcluster, "WIDTH_MAX"=w520:string)  [unwired: 1 out]
        }
        frame "WIDTH_MIN" {
          n131 = property class="PRM"(reference=w522, error in=w525) -> (error out=w523:errorcluster, "WIDTH_MIN"=w524:string)  [unwired: 1 out]
        }
        frame "WRITE_FILE_FFS" {
          n132 = property class="PRM"(reference=w526, error in=w529) -> (error out=w527:errorcluster, "WRITE_FILE_FFS"=w528:string)  [unwired: 1 out]
        }
        frame "ACQ_BUFFER_SIZE_UNIT" {
          n133 = property class="PRM"(reference=w533, error in=w532) -> (error out=w531:errorcluster, "ACQ_BUFFER_SIZE_UNIT"=w530:string)  [unwired: 1 out]
        }
        frame "ACQ_TRANSPORT_BUFFER_COMMIT" {
          n134 = property class="PRM"(reference=w537, error in=w536) -> (error out=w535:errorcluster, "ACQ_TRANSPORT_BUFFER_COMMIT"=w534:string)  [unwired: 1 out]
        }
        frame "AEAG_ROI_HEIGHT" {
          n135 = property class="PRM"(reference=w541, error in=w540) -> (error out=w539:errorcluster, "AEAG_ROI_HEIGHT"=w538:string)  [unwired: 1 out]
        }
        frame "AEAG_ROI_OFFSET_X" {
          n136 = property class="PRM"(reference=w545, error in=w544) -> (error out=w543:errorcluster, "AEAG_ROI_OFFSET_X"=w542:string)  [unwired: 1 out]
        }
        frame "AEAG_ROU_OFFSET_Y" {
          n137 = property class="PRM"(reference=w549, error in=w548) -> (error out=w547:errorcluster, "AEAG_ROI_OFFSET_Y"=w546:string)  [unwired: 1 out]
        }
        frame "AEAG_ROI_WIDTH" {
          n138 = property class="PRM"(reference=w553, error in=w552) -> (error out=w551:errorcluster, "AEAG_ROI_WIDTH"=w550:string)  [unwired: 1 out]
        }
        frame "API_CONTEXT_LIST" {
          n139 = property class="PRM"(reference=w557, error in=w556) -> (error out=w555:errorcluster, "API_CONTEXT_LIST"=w554:string)  [unwired: 1 out]
        }
        frame "BINNING_HORIZONTAL" {
          n140 = property class="PRM"(reference=w561, error in=w560) -> (error out=w559:errorcluster, "BINNING_HORIZONTAL"=w558:string)  [unwired: 1 out]
        }
        frame "BINNING_SELECTOR" {
          n141 = property class="PRM"(reference=w565, error in=w564) -> (error out=w563:errorcluster, "BINNING_SELECTOR"=w562:string)  [unwired: 1 out]
        }
        frame "BINNING_VERTICAL" {
          n142 = property class="PRM"(reference=w569, error in=w568) -> (error out=w567:errorcluster, "BINNING_VERTICAL"=w566:string)  [unwired: 1 out]
        }
        frame "COLUMN_FPN_CORRECTION" {
          n143 = property class="PRM"(reference=w573, error in=w572) -> (error out=w571:errorcluster, "COLUMN_FPN_CORRECTION"=w570:string)  [unwired: 1 out]
        }
        frame "COUNTER_SELECTOR" {
          n144 = property class="PRM"(reference=w577, error in=w576) -> (error out=w575:errorcluster, "COUNTER_SELECTOR"=w574:string)  [unwired: 1 out]
        }
        frame "COUNTER_VALUE" {
          n145 = property class="PRM"(reference=w581, error in=w580) -> (error out=w579:errorcluster, "COUNTER_VALUE"=w578:string)  [unwired: 1 out]
        }
        frame "DECIMATION_HORIZONTAL" {
          n146 = property class="PRM"(reference=w585, error in=w584) -> (error out=w583:errorcluster, "DECIMATION_HORIZONTAL"=w582:string)  [unwired: 1 out]
        }
        frame "DECIMATION_SELECTOR" {
          n147 = property class="PRM"(reference=w589, error in=w588) -> (error out=w587:errorcluster, "DECIMATION_SELECTOR"=w586:string)  [unwired: 1 out]
        }
        frame "DECIMATION_VERTICAL" {
          n148 = property class="PRM"(reference=w593, error in=w592) -> (error out=w591:errorcluster, "DECIMATION_VERTICAL"=w590:string)  [unwired: 1 out]
        }
        frame "DEVICE_ID" {
          n149 = property class="PRM"(reference=w597, error in=w596) -> (error out=w595:errorcluster, "DEVICE_ID"=w594:string)  [unwired: 1 out]
        }
        frame "DEVICE_LOCATION_PATH" {
          n150 = property class="PRM"(reference=w601, error in=w600) -> (error out=w599:errorcluster, "DEVICE_LOCATION_PATH"=w598:string)  [unwired: 1 out]
        }
        frame "DEVICE_MANIFEST" {
          n151 = property class="PRM"(reference=w605, error in=w604) -> (error out=w603:errorcluster, "DEVICE_MANIFEST"=w602:string)  [unwired: 1 out]
        }
        frame "DEVICE_RESET" {
          n152 = property class="PRM"(reference=w609, error in=w608) -> (error out=w607:errorcluster, "DEVICE_RESET"=w606:string)  [unwired: 1 out]
        }
        frame "DEVICE_SENS_SN" {
          n153 = property class="PRM"(reference=w613, error in=w612) -> (error out=w611:errorcluster, "DEVICE_SENS_SN"=w610:string)  [unwired: 1 out]
        }
        frame "EXPOSURE_BURST_COUNT" {
          n154 = property class="PRM"(reference=w617, error in=w616) -> (error out=w615:errorcluster, "EXPOSURE_BURST_COUNT"=w614:string)  [unwired: 1 out]
        }
        frame "FFS_ACCESS_KEY" {
          n155 = property class="PRM"(reference=w621, error in=w620) -> (error out=w619:errorcluster, "FFS_ACCESS_KEY"=w618:string)  [unwired: 1 out]
        }
        frame "GAIN_SELECTOR" {
          n156 = property class="PRM"(reference=w625, error in=w624) -> (error out=w623:errorcluster, "GAIN_SELECTOR"=w622:string)  [unwired: 1 out]
        }
        frame "HW_REVISION" {
          n157 = property class="PRM"(reference=w629, error in=w628) -> (error out=w627:errorcluster, "HW_REVISION"=w626:string)  [unwired: 1 out]
        }
        frame "IMAGE_BLACK_LEVEL" {
          n158 = property class="PRM"(reference=w633, error in=w632) -> (error out=w631:errorcluster, "IMAGE_BLACK_LEVEL"=w630:string)  [unwired: 1 out]
        }
        frame "IMAGE_DATA_BIT_DEPTH" {
          n159 = property class="PRM"(reference=w637, error in=w636) -> (error out=w635:errorcluster, "IMAGE_DATA_BIT_DEPTH"=w634:string)  [unwired: 1 out]
        }
        frame "IMAGE_DATA_FORMAT_RGB32_ALPHA" {
          n160 = property class="PRM"(reference=w641, error in=w640) -> (error out=w639:errorcluster, "IMAGE_DATA_FORMAT_RGB32_ALPHA"=w638:string)  [unwired: 1 out]
        }
        frame "IMAGE_PAYLOAD_SIZE" {
          n161 = property class="PRM"(reference=w645, error in=w644) -> (error out=w643:errorcluster, "IMAGE_PAYLOAD_SIZE"=w642:string)  [unwired: 1 out]
        }
        frame "LENS_APERTURE_VALUE" {
          n162 = property class="PRM"(reference=w649, error in=w648) -> (error out=w647:errorcluster, "LENS_APERTURE_VALUE"=w646:string)  [unwired: 1 out]
        }
        frame "LENS_FEATURE" {
          n163 = property class="PRM"(reference=w653, error in=w652) -> (error out=w651:errorcluster, "LENS_FEATURE"=w650:string)  [unwired: 1 out]
        }
        frame "LENS_FEATURE_SELECTOR" {
          n164 = property class="PRM"(reference=w657, error in=w656) -> (error out=w655:errorcluster, "LENS_FEATURE_SELECTOR"=w654:string)  [unwired: 1 out]
        }
        frame "LENS_FOCAL_LENGTH" {
          n165 = property class="PRM"(reference=w661, error in=w660) -> (error out=w659:errorcluster, "LENS_FOCAL_LENGTH"=w658:string)  [unwired: 1 out]
        }
        frame "LENS_FOCUS_DISTANCE" {
          n166 = property class="PRM"(reference=w665, error in=w664) -> (error out=w663:errorcluster, "LENS_FOCUS_DISTANCE"=w662:string)  [unwired: 1 out]
        }
        frame "LENS_FOCUS_MOVE" {
          n167 = property class="PRM"(reference=w669, error in=w668) -> (error out=w667:errorcluster, "LENS_FOCUS_MOVE"=w666:string)  [unwired: 1 out]
        }
        frame "LENS_FOCUS_MOVEMENT_VALUE" {
          n168 = property class="PRM"(reference=w673, error in=w672) -> (error out=w671:errorcluster, "LENS_FOCUS_MOVEMENT_VALUE"=w670:string)  [unwired: 1 out]
        }
        frame "LENS_MODE" {
          n169 = property class="PRM"(reference=w677, error in=w676) -> (error out=w675:errorcluster, "LENS_MODE"=w674:string)  [unwired: 1 out]
        }
        frame "OUTPUT_DATA_PACKING_TYPE" {
          n170 = property class="PRM"(reference=w681, error in=w680) -> (error out=w679:errorcluster, "OUTPUT_DATA_PACKING_TYPE"=w678:string)  [unwired: 1 out]
        }
        frame "SENSOR_CLOCK_FREQ_HZ" {
          n171 = property class="PRM"(reference=w685, error in=w684) -> (error out=w683:errorcluster, "SENSOR_CLOCK_FREQ_HZ"=w682:string)  [unwired: 1 out]
        }
        frame "SENSOR_CLOCK_FREQ_INDEX" {
          n172 = property class="PRM"(reference=w689, error in=w688) -> (error out=w687:errorcluster, "SENSOR_CLOCK_FREQ_INDEX"=w686:string)  [unwired: 1 out]
        }
        frame "SENSOR_FEATURE_SELECTOR" {
          n173 = property class="PRM"(reference=w693, error in=w692) -> (error out=w691:errorcluster, "SENSOR_FEATURE_SELECTOR"=w690:string)  [unwired: 1 out]
        }
        frame "SENSOR_FEATURE_VALUE" {
          n174 = property class="PRM"(reference=w697, error in=w696) -> (error out=w695:errorcluster, "SENSOR_FEATURE_VALUE"=w694:string)  [unwired: 1 out]
        }
        frame "SENSOR_OUTPUT_CHANNEL_COUNT" {
          n175 = property class="PRM"(reference=w701, error in=w700) -> (error out=w699:errorcluster, "SENSOR_OUTPUT_CHANNEL_COUNT"=w698:string)  [unwired: 1 out]
        }
        frame "TRANSPORT_PIXEL_FORMAT" {
          n176 = property class="PRM"(reference=w705, error in=w704) -> (error out=w703:errorcluster, "TRANSPORT_PIXEL_FORMAT"=w702:string)  [unwired: 1 out]
        }
        frame "TS_RST_MODE" {
          n177 = property class="PRM"(reference=w709, error in=w708) -> (error out=w707:errorcluster, "TS_RST_MODE"=w706:string)  [unwired: 1 out]
        }
        frame "TS_RST_SOURCE" {
          n178 = property class="PRM"(reference=w713, error in=w712) -> (error out=w711:errorcluster, "TS_RST_SOURCE"=w710:string)  [unwired: 1 out]
        }
        frame "SENS_DEFECTS_CORR_LIST_SELECTOR" {
          n179 = property class="PRM"(reference=w714, error in=w715) -> (error out=w716:errorcluster, "SENS_DEFECTS_CORR_LIST_SELECTOR"=w717:string)  [unwired: 1 out]
        }
        frame "SENS_DEFECTS_CORR" {
          n180 = property class="PRM"(reference=w718, error in=w721) -> (error out=w720:errorcluster, "SENS_DEFECTS_CORR"=w719:string)  [unwired: 1 out]
        }
        frame "SENS_DEFECTS_CORR_LIST_CONTENT" {
          n181 = property class="PRM"(reference=w722, error in=w725) -> (error out=w724:errorcluster, "SENS_DEFECTS_CORR_LIST_CONTENT"=w723:string)  [unwired: 1 out]
        }
        frame "DEVICE_UNIT_SELECTOR" {
          n182 = property class="PRM"(reference=w728, error in=w729) -> (error out=w727:errorcluster, "DEVICE_UNIT_SELECTOR"=w726:string)  [unwired: 1 out]
        }
        frame "DEVICE_UNIT_REGISTER_SELECTOR" {
          n183 = property class="PRM"(reference=w732, error in=w733) -> (error out=w731:errorcluster, "DEVICE_UNIT_REGISTER_SELECTOR"=w730:string)  [unwired: 1 out]
        }
        frame "DEVICE_UNIT_REGISTER_VALUE" {
          n184 = property class="PRM"(reference=w736, error in=w737) -> (error out=w735:errorcluster, "DEVICE_UNIT_REGISTER_VALUE"=w734:string)  [unwired: 1 out]
        }
      }
    }
    frame Error {
    }
  }
  "error out" <- w2
  "ParameterString" <- w1
  "PRM OUT" <- "PRM"
